vi "Update ColHdrs[].vi"(8 "error in (no error)":errorcluster, 9 "Active Cell:Cell Justification":enum16{"Left", "Center", "Right"}(ring), 10 "Column Header Strings[]":string[](array[string]), 11 "MCLB_Lib in":refnum<class "MCLB_Lib.lvclass">) -> (0 "error out":errorcluster, 3 "MCLB_Lib out":refnum<class "MCLB_Lib.lvclass">)   [LabVIEW 2020, in "MCLB_Lib.lvclass"]
uses:
  MCLB_Lib.lvclass
  MCLB_Lib.lvclass/MCLB_Lib.ctl
  <vilib>/Utility/miscctls.llb/LVRowAndColumnTypeDef.ctl
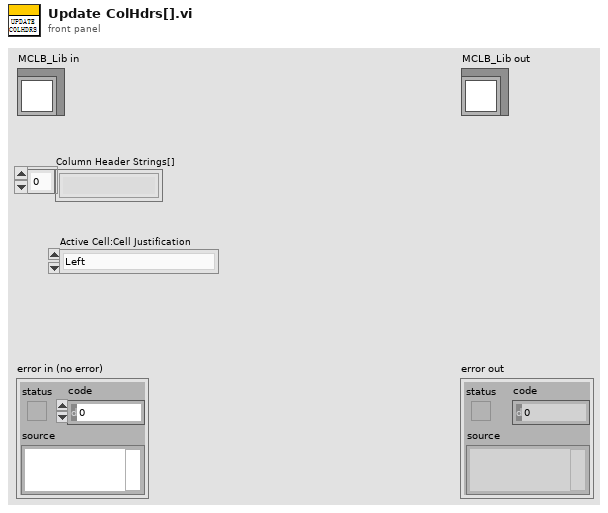
[diagram p1: front panel]
types:
  T1 = typedef "LVRowAndColumnTypeDef.ctl" = cluster{"Row":i32, "Column":i32}
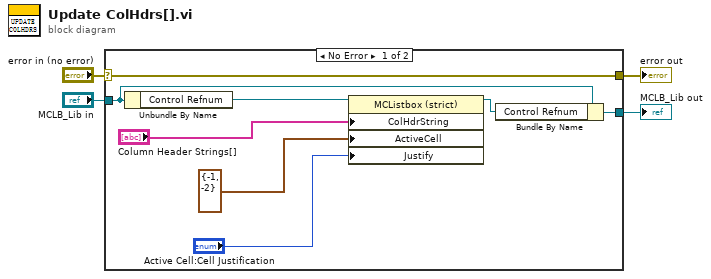
[diagram p0: block diagram]
diagram:
  n1 = case shown="No Error" "error in (no error)" {
    selector: "error in (no error)" -> [w12 w14]
    tunnel: [w12 w14] -> w3
    tunnel: [w9 w13] -> w1
    tunnel: "MCLB_Lib in" -> [w8 w13]
    frame No Error {
      n2 = Unbundle By Name(w8) -> ("Control Refnum"=w10:refnum<vi>)
      n3 = property class="MCListbox (strict)"(reference=w10, "ColHdrString"="Column Header Strings[]", "ActiveCell"=T1 {"Row"=-1, "Column"=-2} ("Active Cell:Active Cell"), "Justify"="Active Cell:Cell Justification") -> (reference out=w11:refnum<vi>)  [unwired: 1 in, 1 out]
      n4 = Bundle By Name(cluster=w8, "Control Refnum"=w11) -> (w9:refnum<class "MCLB_Lib.lvclass">)
    }
    frame Error {
    }
  }
  "error out" <- w3
  "MCLB_Lib out" <- w1
